vi "ReadSweepConfigurationExample.vi"   [LabVIEW 2016, in "SweepControl.lvclass"]
uses:
  SweepControl/SweepControl.lvclass
  SweepControl/Typedefs/Enum - Experiments.ctl
  SweepControl/Typedefs/Continuous B Sweep Configuration--Cluster.ctl
  SweepControl/Typedefs/Enum - Priority.ctl
  SweepControl/Typedefs/Enum - Action.ctl
  SweepControl/Typedefs/Cluster - ScanControl.ctl
  SweepControl/Typedefs/ScanControl.ctl
  SweepControl/Typedefs/Cluster - ScanParamters.ctl
  SweepControl/Typedefs/ScanParamters.ctl
  SweepControl/Typedefs/Sweep Control Configuration--Cluster.ctl
  LockinVsg Configuration--Cluster.ctl
  Transport.lvclass
panel:
  # "See block diagram for example of how to use ReadSweepConfigurationFile.vi"
types:
  T1 = typedef "Transport.lvclass/LockinVsg Configuration--Cluster.ctl" = cluster{"Vsg Values":dbl[]}
  T2 = typedef "SweepControl.lvclass/Sweep Control Configuration--Cluster.ctl" = cluster{"Scan control":T3, "Scan parameters":T7, "Experiment":T9}
  T3 = typedef "SweepControl.lvclass/ScanControl.ctl" = T4[]
  T4 = typedef "SweepControl.lvclass/Cluster - ScanControl.ctl" = cluster{"Priority":T5, "Scan name":T6}
  T5 = typedef "SweepControl.lvclass/Enum - Priority.ctl" = enum16{"Priority 0", "Priority 1", "Priority 2", "Priority 3", "Priority 4", "Priority 5"}
  T6 = typedef "SweepControl.lvclass/Enum - Action.ctl" = enum16{"OFF", "DSA_Vamp", "DSA_freq", "DSA_Vsg1", "DSA_Vsg2", "DSA_Vsg3", "DAQ_Vbg", "B_Field", "Humidity", "Temp", "MW_freq1", "MW_freq2", "MW_amplitude1", "MW_amplitude2"}
  T7 = typedef "SweepControl.lvclass/ScanParamters.ctl" = T8[]
  T8 = typedef "SweepControl.lvclass/Cluster - ScanParamters.ctl" = cluster{"Start":dbl, "End":dbl, "Step":dbl, "Rate":dbl, "wait (ms)":u32, "Address":string, "channel":i32}
  T9 = typedef "SweepControl.lvclass/Enum - Experiments.ctl" = enum16{"IV", "Lockin_time", "Lockin_Vsg", "Lockin (experimental)", "Lockin_Vsg_JKISM"}
  T10 = typedef "SweepControl.lvclass/Continuous B Sweep Configuration--Cluster.ctl" = cluster{"B field values":dbl[], "Experiment":T9}
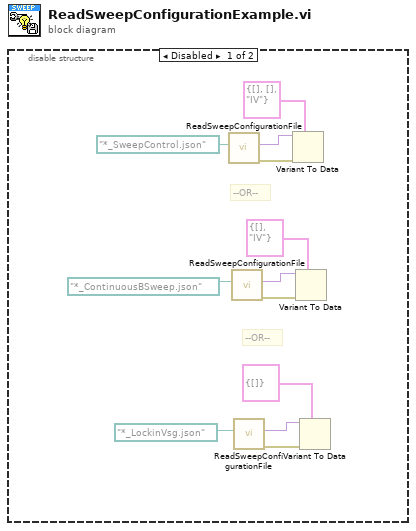
[diagram p0: block diagram]
diagram:
  n1 = disable-structure shown="Disabled" {
    frame Disabled {
      # "--OR--"
      # "--OR--"
      n2 = call "ReadSweepConfigurationFile.vi"("Path"=path "*_SweepControl.json") -> ("error out"=w9:errorcluster, "Data"=w5:variant)  [unwired: 8 in, 1 out]
      n3 = call "ReadSweepConfigurationFile.vi"("Path"=path "*_ContinuousBSweep.json") -> ("error out"=w6:errorcluster, "Data"=w4:variant)  [unwired: 8 in, 1 out]
      n4 = call "ReadSweepConfigurationFile.vi"("Path"=path "*_LockinVsg.json") -> ("error out"=w8:errorcluster, "Data"=w7:variant)  [unwired: 8 in, 1 out]
      n5 = Variant To Data(error in=w9, type=T2 {"Scan control"=[], "Scan parameters"=[], "Experiment"=enum."IV"} ("SweepControl"), Variant=w5) -> ()  [unwired: 2 out]
      n6 = Variant To Data(error in=w6, type=T10 {"B field values"=[], "Experiment"=enum."IV"} ("ContinuousBSweep"), Variant=w4) -> ()  [unwired: 2 out]
      n7 = Variant To Data(error in=w8, type=T1 {"Vsg Values"=[]} ("LockinVsg Sweep"), Variant=w7) -> ()  [unwired: 2 out]
    }
    frame Enabled {
    }
  }
